vi "Generate Error Code.vi"(7 "Warning? (False)":bool, 8 "error in":errorcluster, 10 "Error Details":string, 11 "Error Code (-9999)":i32(ring)=-9999 items=["No error", "Argument error", "Memory is full", "Out of zone", "End of file", "File already open", "Generic file I/O error", "File not found", "File permission error", "Disk is full", "Duplicate path", "Too many files open", "System feature not enabled", "Resource file not found", "Cannot add resource", "Resource not found", "Image not found", "Image memory error", "Pen does not exist", "Config type invalid", "Config token not found", "Config parse error", "Config memory error", "Bad external code format", "Bad external code offset", "External code not present", "Null window", "Destroy window error", "Null menu", "Print aborted", "Bad print record", "Print driver error", "Windows error during printing", "Memory error during printing", "Print dialog error", "Generic print error", "Invalid device refnum", "Device not found", "Device parameter error", "Device unit error", "Cannot open device", "Device call aborted", "Generic error", "Cancelled by user", "Object ID too low", "Object ID too high", "Object not in heap", "Unknown heap", "Unknown object (invalid DefProc)", "Unknown object (DefProc not in table)", "Message out of range", "Invalid (null) method", "Unknown message", "Manager call not supported", "Bad address", "Network operation in progress", "Network operation timed out", "Connection is busy", "Network attribute not supported", "Network error", "Address in use", "System out of memory", "Connection aborted", "Connection refused", "Not connected", "Already connected", "Connection closed", "Initialization error (interapplication manager)", "Bad occurrence", "Wait on unbound occurrence handler", "Occurrence queue overflow", "Datalog type conflict", "Unused", "Unrecognized type (interapplication manager)", "Memory corrupt", "Failed to make temporary DLL", "Old CIN version", "Drag socket not found", "Failed to load drop-object", "Failed to register OLE object", "Failed to release OLE object", "Format specifier type mismatch", "Unknown format specifier", "Too few format specifiers", "Too many format specifiers", "Scan failed", "Newer CIN version", "OLE Convert", "Runtime menu error", "Password tampered", "Unknown error code"]) -> (0 "error out":errorcluster)   [LabVIEW 2011]
doc: "Generates an error with the passed in error number, details.\n\n\nVersion 1.1 - 6/1/2010\n\nPhaeron, Inc.\nwww.phaeron.com\ninfo@phaeron.com"
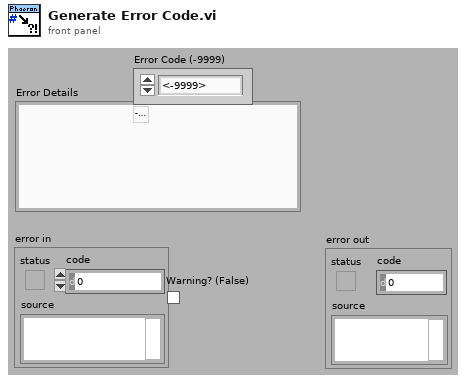
[diagram p1: front panel]
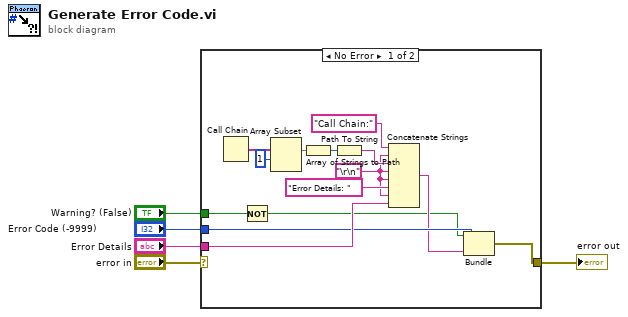
[diagram p0: block diagram]
diagram:
  n1 = case shown="No Error" "error in" {
    selector: "error in" -> [_ w20]
    tunnel: "Error Details" -> [w13 _]
    tunnel: [w9 w20] -> w3
    tunnel: "Warning? (False)" -> [w12 _]
    tunnel: "Error Code (-9999)" -> [w11 _]
    frame No Error {
      w7 = "\r\n"
      n2 = Call Chain() -> (call chain=w18:string[])
      n3 = Not(x=w12) -> (.not. x?=w6:bool)
      n4 = Array Subset(array=w18, index=1) -> (w17:string[])  [unwired: 1 in]
      n5 = Array of Strings to Path(0:w17) -> (2:w16:path)  [unwired: 1 out]
      n6 = Path To String(path=w16) -> (string=w14:string)
      n7 = Concatenate Strings("Call Chain:" ("string"), w7, w14, w7, w7, "Error Details: " ("string"), w7, w13) -> (w10:string)
      n8 = Bundle(w6, "Error Code (-9999)"=w11, w10) -> (w9:cluster{bool, "Error Code (-9999)":i32, string})  [unwired: 1 out]
    }
    frame Error {
    }
  }
  "error out" <- w3
